vi "Hex to Str Hex.vi"(11 "String":string) -> (3 "hex integer string":string)   [LabVIEW 2018]
panel:
  out "*(type *) &x":i32
  # "2022-08-31"
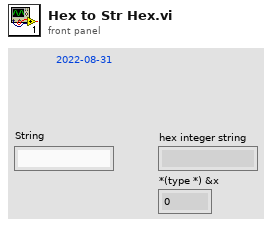
[diagram p1: front panel]
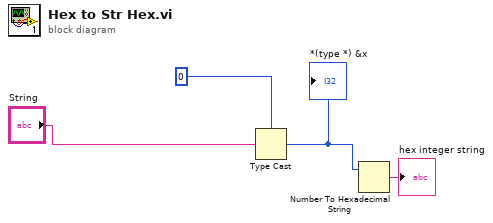
[diagram p0: block diagram]
diagram:
  n1 = Type Cast(type=0, x="String") -> (*(type *) &x=w2:i32)
  "*(type *) &x" <- w2
  n2 = Number To Hexadecimal String(2:w2) -> (0:→"hex integer string":string)  [unwired: 1 in]
